vi "USRP Calculate Power Spectrum.vi"(0 "waveform":waveform(cdb)) -> (4 "power spectrum (dBm)":cluster{"f0":dbl, "df":dbl, "magnitude":dbl[]})   [LabVIEW 2016]
doc: "Calculates the power spectrum from the I/Q data."
uses:
  <vilib>/measure/maspectr.llb/FFT Power Spectrum and PSD for 1 Chan (CDB).vi
  <vilib>/measure/NI_MAPro.lvlib
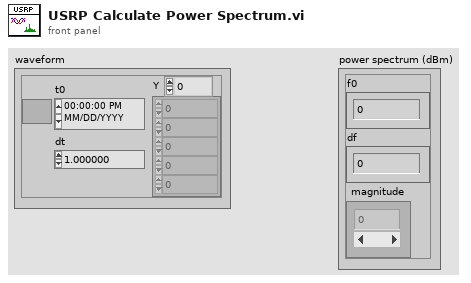
[diagram p1: front panel]
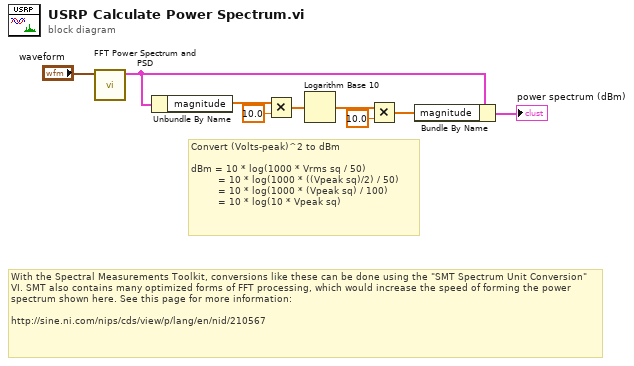
[diagram p0: block diagram]
diagram:
  # "With the Spectral Measurements Toolkit, conversions like these can be done using the \"SMT Spectrum Unit Conversion\" VI. SMT also contains many optimized forms of FFT processing, which would increase the speed of forming the power spectrum shown here. See this page for more information: \n\nhttp://sine.ni.com/nips/cds/view/p/lang/en/nid/210567"
  # "Convert (Volts-peak)^2 to dBm\n\ndBm = 10 * log(1000 * Vrms sq / 50)\n         = 10 * log(1000 * ((Vpeak sq)/2) / 50) \n         = 10 * log(1000 * (Vpeak sq) / 100) \n         = 10 * log(10 * Vpeak sq)"
  n1 = call-poly <vilib>:"FFT Power Spectrum and PSD.vi"("time signal"="waveform") -> ("Power Spectrum / PSD"=w9:cluster{"f0":dbl, "df":dbl, "magnitude":dbl[]})  [unwired: 7 in, 3 out]
  n2 = Unbundle By Name(w9) -> ("magnitude"=w5:dbl[])
  n3 = Multiply(x=w5, y=10.0) -> (x*y=w4:dbl[])
  n4 = Logarithm Base 10(1:w4) -> (0:w3:dbl[])
  n5 = Multiply(x=w3, y=10.0) -> (x*y=w2:dbl[])
  n6 = Bundle By Name(cluster=w9, "magnitude"=w2) -> (→"power spectrum (dBm)":cluster{"f0":dbl, "df":dbl, "magnitude":dbl[]})
